vi "convert sensor voltage to real measurements.vi"(9 "Input Variables and Slopes":T2={"Total Volume"=0.0, "String Pot Slope"=0.0, "Flow Slope"=0.0, "Up Hole Pressure Slope"=0.0, "Depth to Water Table"=0.0, "Atmospheric Pressure"=0.0, "DH Pressure Trans Slope"=0.0, "DH Pressure Offset"=0.0, "Up Hole  Pressure Offset"=0.0, "Aux 1 Slope"=1.6619999408721924, "Aux 2 Slope"=39.040000915527344, "Aux 3 Slope"=48.27000045776367, "Aux 1 Offset"=0.0, "Aux 2 Offset"=0.0, "Aux 3 Offset"=0.0, "String Pot Offset"=0.0, "Flow Offset"=0.0, "Reservoir Pressure"=0.0, "Height of Sample Box"=0.0, "Feet of Stainless "=0} {"Feet of Stainless" format="%.2f"; "Height of Sample Box" format="%.2f"; "Reservoir Pressure" format="%.2f"; "Flow Offset" format="%.2f"; "String Pot Offset" format="%.2f"; "Aux 3 Offset" format="%.2f"; "Aux 2 Offset" format="%.2f"; "Aux 1 Offset" format="%.2f"; "Aux 3 Slope" format="%.2f"; "Aux 2 Slope" format="%.2f"; "Aux 1 Slope" format="%.2f"; "Up Hole  Pressure Offset" format="%.2f"; "DH Pressure Offset" format="%.2f"; "DH Pressure Trans Slope" format="%.2f"; "Atmospheric Pressure" format="%.2f"; "Depth to Water Table" format="%.2f"; "Up Hole Pressure Slope" format="%.2f"; "Flow Slope" format="%.2f"; "String Pot Slope" format="%.2f"; "Total Volume" format="%.2f"}, 10 "Sensor  Real Measurements in":T1, 11 "Sensor Cluster":T1) -> (3 "Sensor  Real Measurements out":T1)   [LabVIEW 2016]
uses:
  controls/MCC DAQ Readings.ctl
  Control 2.ctl
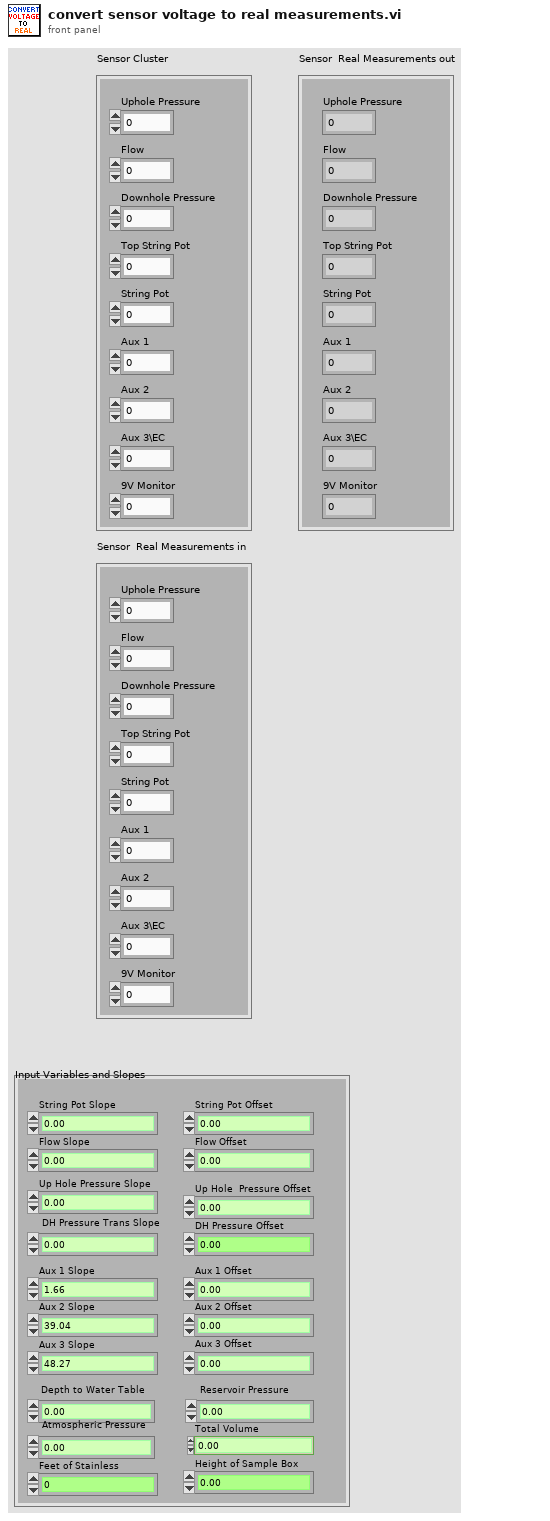
[diagram p1: front panel]
types:
  T1 = typedef "MCC DAQ Readings.ctl" = cluster{"Uphole Pressure":dbl, "Flow":dbl, "Downhole Pressure":dbl, "Top String Pot":dbl, "String Pot":dbl, "Aux 1":dbl, "Aux 2":dbl, "Aux 3\\EC":dbl, "9V Monitor":dbl}
  T2 = typedef "Control 2.ctl" = cluster{"Total Volume":dbl, "String Pot Slope":dbl, "Flow Slope":dbl, "Up Hole Pressure Slope":dbl, "Depth to Water Table":dbl, "Atmospheric Pressure":dbl, "DH Pressure Trans Slope":dbl, "DH Pressure Offset":dbl, "Up Hole  Pressure Offset":dbl, "Aux 1 Slope":dbl, "Aux 2 Slope":dbl, "Aux 3 Slope":dbl, "Aux 1 Offset":dbl, "Aux 2 Offset":dbl, "Aux 3 Offset":dbl, "String Pot Offset":dbl, "Flow Offset":dbl, "Reservoir Pressure":dbl, "Height of Sample Box":dbl, "Feet of Stainless ":i32}
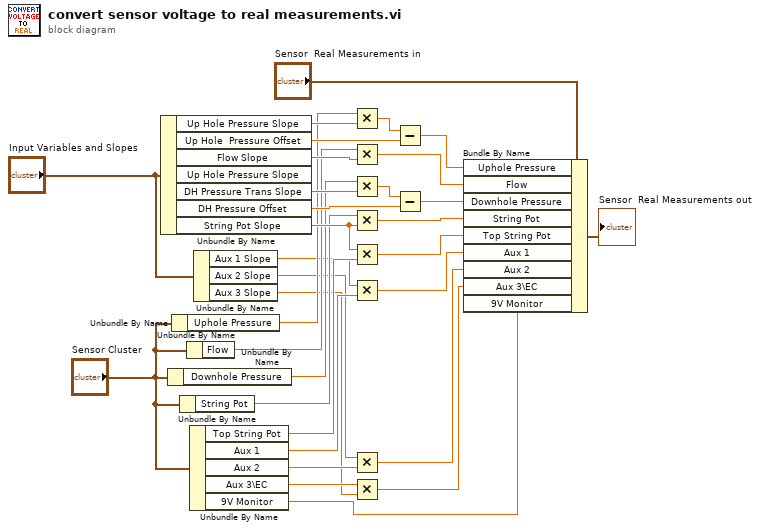
[diagram p0: block diagram]
diagram:
  n1 = Unbundle By Name("Input Variables and Slopes") -> ("Up Hole Pressure Slope"=w15:dbl, "Up Hole  Pressure Offset"=w18:dbl, "Flow Slope"=w20:dbl, "DH Pressure Trans Slope"=w23:dbl, "DH Pressure Offset"=w25:dbl, "String Pot Slope"=w29:dbl)  [unwired: 1 out]
  n2 = Unbundle By Name("Sensor Cluster") -> ("Downhole Pressure"=w22:dbl)
  n3 = Unbundle By Name("Sensor Cluster") -> ("Uphole Pressure"=w14:dbl)
  n4 = Unbundle By Name("Sensor Cluster") -> ("String Pot"=w27:dbl)
  n5 = Unbundle By Name("Sensor Cluster") -> ("Flow"=w19:dbl)
  n6 = Unbundle By Name("Sensor Cluster") -> ("Top String Pot"=w30:dbl, "Aux 1"=w11:dbl, "Aux 2"=w10:dbl, "Aux 3\\EC"=w9:dbl, "9V Monitor"=w1:dbl)
  n7 = Unbundle By Name("Input Variables and Slopes") -> ("Aux 1 Slope"=w4:dbl, "Aux 2 Slope"=w3:dbl, "Aux 3 Slope"=w2:dbl)
  n8 = Multiply(x=w14, y=w15) -> (x*y=w17:dbl)
  n9 = Multiply(x=w19, y=w20) -> (x*y=w21:dbl)
  n10 = Multiply(x=w22, y=w23) -> (x*y=w24:dbl)
  n11 = Multiply(x=w27, y=w29) -> (x*y=w28:dbl)
  n12 = Multiply(x=w29, y=w30) -> (x*y=w31:dbl)
  n13 = Multiply(x=w4, y=w11) -> (x*y=w8:dbl)
  n14 = Multiply(x=w3, y=w10) -> (x*y=w7:dbl)
  n15 = Multiply(x=w9, y=w2) -> (x*y=w6:dbl)
  n16 = Subtract(x=w17, y=w18) -> (x-y=w16:dbl)
  n17 = Subtract(x=w24, y=w25) -> (x-y=w26:dbl)
  n18 = Bundle By Name(cluster="Sensor  Real Measurements in", "Uphole Pressure"=w16, "Flow"=w21, "Downhole Pressure"=w26, "String Pot"=w28, "Top String Pot"=w31, "Aux 1"=w8, "Aux 2"=w7, "Aux 3\\EC"=w6, "9V Monitor"=w1) -> (→"Sensor  Real Measurements out":T1)
